vi "ShooterSpeedChoose.vi"(7 "DRIVER OFF":bool, 8 "3pt Key Shot Button":bool, 9 "2pt Key Shot Button":bool, 10 "Long Shot Button":bool, 11 "Warm Button":bool) -> (3 "Shooter Speed":T1(ring))   [LabVIEW 2012]
uses:
  2013 Ultimate Ascent/Robot Global Data.vi
panel:
  # "Operator\nButton 1: Shooter Warm\nButton 2: Shooter Long Shot\nButton 3: Shooter 2pt Key Shot\nButton 4: Shooter normal key shot"
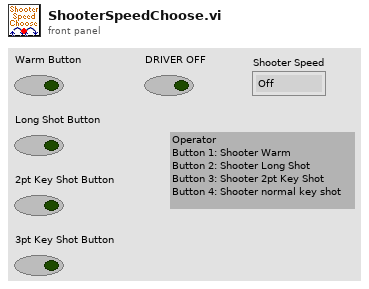
[diagram p1: front panel]
types:
  T1 = enum16{"Off", "2pt Key Shot", "3pt Key Shot", "Back Shot", "Fender Shot"}
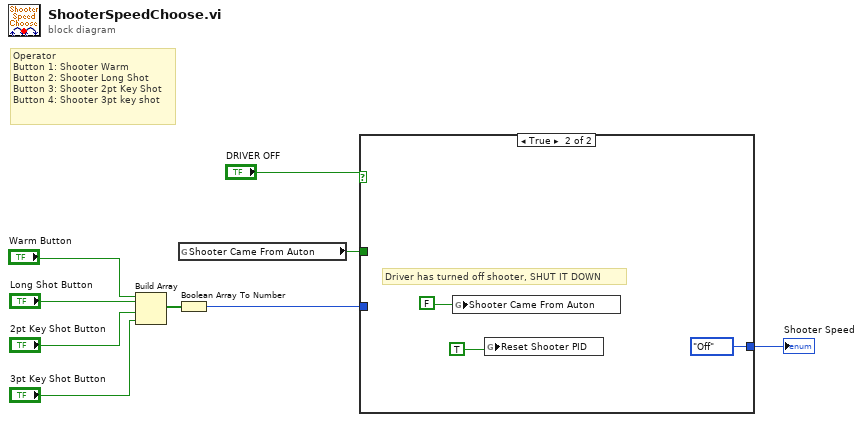
[diagram p0: block diagram]
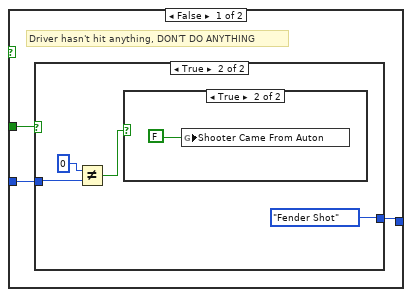
[diagram p2: hidden frame]
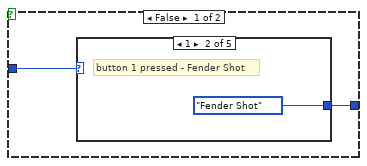
[diagram p3: hidden frame]
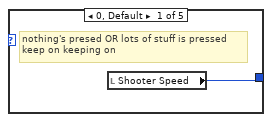
[diagram p4: hidden frame]
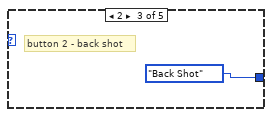
[diagram p5: hidden frame]
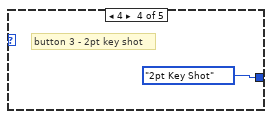
[diagram p6: hidden frame]
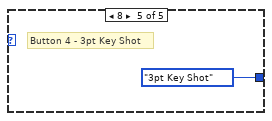
[diagram p7: hidden frame]
diagram:
  # "Operator\nButton 1: Shooter Warm\nButton 2: Shooter Long Shot\nButton 3: Shooter 2pt Key Shot\nButton 4: Shooter 3pt key shot"
  n1 = Build Array("Warm Button", "Long Shot Button", "2pt Key Shot Button", "3pt Key Shot Button") -> (w9:bool[])
  n2 = global read "Robot Global Data.vi" "Shooter Came From Auton"() -> (w1:bool)
  n3 = Boolean Array To Number(Boolean array=w9) -> (number=w2:u32)
  n4 = case shown="True" "DRIVER OFF" {
    tunnel: w2 -> [w11 _]
    tunnel: [w12 T1."Off" ("Shooter Speed")] -> w3
    tunnel: w1 -> [w10 _]
    frame False {
      # "Driver hasn't hit anything, DON'T DO ANYTHING"
      n5 = case shown="True" w10 {
        tunnel: [w14 T1."Fender Shot" ("Shooter Speed")] -> w12
        tunnel: w11 -> [w13 w21]
        frame False {
          n6 = case shown="1" w13 {
            tunnel: [w15 T1."Fender Shot" ("Shooter Speed") T1."Back Shot" ("Shooter Speed") T1."2pt Key Shot" ("Shooter Speed") T1."3pt Key Shot" ("Shooter Speed")] -> w14
            frame 0, Default {
              # "nothing's presed OR lots of stuff is pressed\nkeep on keeping on"
              n7 = local read "Shooter Speed"() -> (w15:T1)
            }
            frame 1 {
              # "button 1 pressed - Fender Shot"
            }
            frame 2 {
              # "button 2 - back shot"
            }
            frame 4 {
              # "button 3 - 2pt key shot"
            }
            frame 8 {
              # "Button 4 - 3pt Key Shot"
            }
          }
        }
        frame True {
          n8 = Not Equal?(x=0, y=w21) -> (x != y?=w20:bool)
          n9 = case shown="True" w20 {
            frame False {
            }
            frame True {
              n10 = global write "Robot Global Data.vi" "Shooter Came From Auton"(FALSE) -> ()
            }
          }
        }
      }
    }
    frame True {
      # "Driver has turned off shooter, SHUT IT DOWN"
      n11 = global write "Robot Global Data.vi" "Shooter Came From Auton"(FALSE) -> ()
      n12 = global write "Robot Global Data.vi" "Reset Shooter PID"(TRUE) -> ()
    }
  }
  "Shooter Speed" <- w3
